vi "addParamtToString.vi"(8 "error in (no error)":errorcluster, 9 "param":string, 10 "paramList in":string, 11 "Electrometer in":refnum<class "Electrometer.lvclass">) -> (0 "error out":errorcluster, 2 "paramList out":string, 3 "Electrometer out":refnum<class "Electrometer.lvclass">)   [LabVIEW 2016, in "Electrometer.lvclass"]
uses:
  Electrometer.lvclass
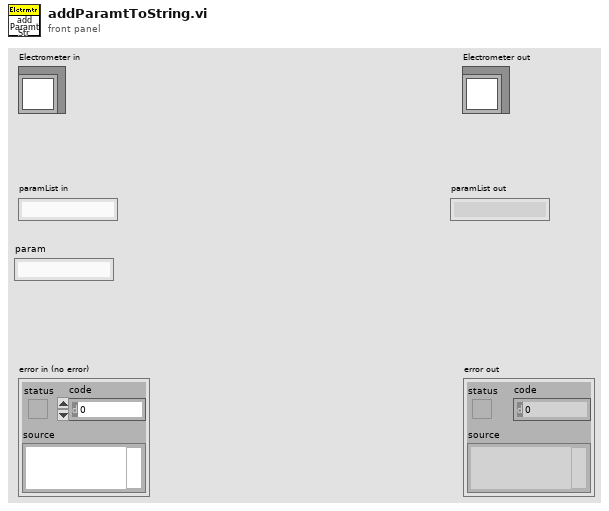
[diagram p1: front panel]
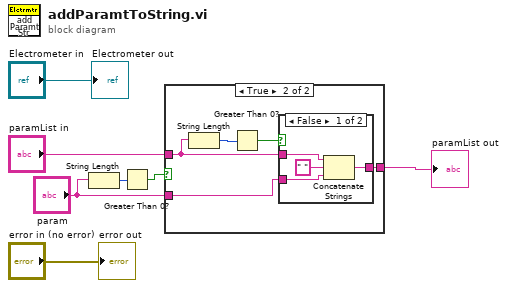
[diagram p0: block diagram]
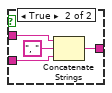
[diagram p3: hidden frame]
diagram:
  n1 = String Length(string="param") -> (length=w2:i32)
  n2 = Greater Than 0?(x=w2) -> (x > 0?=w1:bool)
  n3 = case shown="True" w1 {
    tunnel: "paramList in" -> [w8 w12]
    tunnel: [w8 w10] -> w4
    tunnel: "param" -> [_ w9]
    frame False {
    }
    frame True {
      n4 = String Length(string=w12) -> (length=w13:i32)
      n5 = Greater Than 0?(x=w13) -> (x > 0?=w11:bool)
      n6 = case shown="False" w11 {
        tunnel: w12 -> [w17 w21]
        tunnel: w9 -> [w16 w19]
        tunnel: [w14 w18] -> w10
        frame False {
          n7 = Concatenate Strings(w17, " " ("string"), w16) -> (w14:string)
        }
        frame True {
          n8 = Concatenate Strings(w21, ", " ("string"), w19) -> (w18:string)
        }
      }
    }
  }
  "paramList out" <- w4
  "error out" <- "error in (no error)"
  "Electrometer out" <- "Electrometer in"
